vi "AnalogOutput Interface.vi"(7 "Options":T1={"Waveform type"=enum."sine", "Amplitude (V)"=1.0, "Sample clock (Hz)"=100000.0}, 8 "Eventstring":string, 9 "Duration (ms)":dbl, 10 "Frequency (Hz)":dbl, 11 "Port index":i32) -> (1 "OutputRequest":T2)   [LabVIEW 2015]
doc: "Makes OutputRequest objects compatible with the AnalogOutput output driver.\n\nCurrently only does sine waves\n\nPort index: Port number assigned by the reservation system\nFrequency (Hz): Frequency of sine wave\nDuration (ms): Duration of tone\nEventstring: String to send w/ timestamp, or empty/unwired for no timestamp\nOptions:\n Waveform type: Only one choice: \"sine\"\n Amplitude (V): Peak amplitude in V\n Sample clock (Hz): Rate to sample the signal at"
uses:
  Typedefs/OutputRequest.ctl
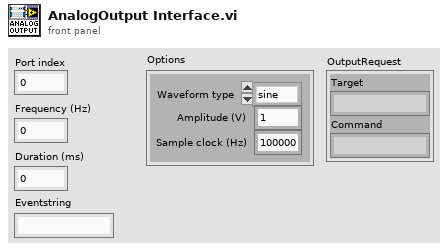
[diagram p1: front panel]
types:
  T1 = cluster{"Waveform type":enum16{"sine"}, "Amplitude (V)":dbl, "Sample clock (Hz)":dbl}
  T2 = typedef "OutputRequest.ctl" = cluster{"Target":string, "Command":string}
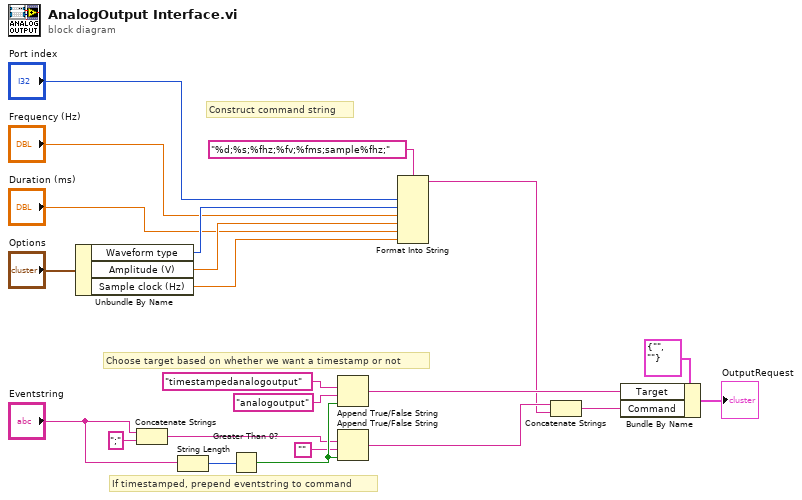
[diagram p0: block diagram]
diagram:
  # "Construct command string"
  # "If timestamped, prepend eventstring to command"
  # "Choose target based on whether we want a timestamp or not"
  n1 = Unbundle By Name("Options") -> ("Waveform type"=w5:enum16{"sine"}, "Amplitude (V)"=w3:dbl, "Sample clock (Hz)"=w1:dbl)
  n2 = Concatenate Strings("Eventstring", ";" ("string")) -> (w13:string)
  n3 = String Length(string="Eventstring") -> (length=w20:i32)
  n4 = Greater Than 0?(x=w20) -> (x > 0?=w14:bool)
  n5 = Append True/False String(1:w14, 2:"analogoutput" ("false string"), 3:"timestampedanalogoutput" ("true string")) -> (0:w17:string)  [unwired: 1 in]
  n6 = Append True/False String(1:w14, 2:"", 3:w13) -> (0:w10:string)  [unwired: 1 in]
  n7 = Format Into String(format string="%d;%s;%fhz;%fv;%fms;sample%fhz;", "Port index", w5, "Frequency (Hz)", w3, "Duration (ms)", w1) -> (resulting string=w7:string)  [unwired: 2 in, 1 out]
  n8 = Concatenate Strings(w10, w7) -> (w11:string)
  n9 = Bundle By Name(cluster=T2 {"Target"="", "Command"=""} ("OutputRequest"), "Target"=w17, "Command"=w11) -> (→"OutputRequest":T2)
